vi "Dependency Change.vi"(5 "object ref in":T3, 8 "error in (no error)":errorcluster, 9 "old values":string[][](array[string]), 10 "Table Change":T2, 11 "Mapping Column in":refnum<class "Mapping Column.lvclass">) -> (0 "error out":errorcluster, 3 "Mapping Column out":refnum<class "Mapping Column.lvclass">)   [LabVIEW 2013, in "Table Manager.lvlib" / "Mapping Column.lvclass"]
uses:
  Mapping Column.lvclass
  Table Manager/object ref.ctl
  <vilib>/NI/DCAF/Tag Editor Core/Configuration Editor/Classes/Engine Parent/Engine Parent Editor Node.lvclass
  <vilib>/NI/DCAF/Tag Editor Core/Configuration Editor/Classes/Module editor node/module editor node.lvclass
  Table Manager/Cell Change.ctl
  <vilib>/NI/Tag Bus/tag/Data Type.ctl
  Mapping Column.lvclass/Mapping Column.ctl
  <vilib>/NI/Tag Bus Module Framework/module configuration/TBM module configuration.lvclass
  <vilib>/NI/Configuration Framework/serializable configuration/NISE_CEF_serializable configuration.lvclass/NISE_CEF_serializable configuration.ctl
  <vilib>/NI/Tag Bus/tag/tag descriptor.lvclass/tag descriptor.ctl
  Read Name Dependecy.vi
  Read Data Type Dependecy.vi
  Read Channel suffix.vi
  Column/Read Call Back VI.vi
  <vilib>/Utility/LVClass/Get LV Class Name.vi
  <vilib>/NI/Configuration Framework/error generator/NISE_error generator.vi
  <vilib>/NI/Module Execution Interface/Engine Configuration/engine configuration.lvclass
  <vilib>/NI/Configuration Framework/serializable configuration/NISE_CEF_serializable configuration.lvclass
  <vilib>/NI/Tag Bus/tag/tag descriptor.lvclass
  Table Manager.lvlib
  Column/Column.lvclass
  Table Manager/Table Manager.lvclass
panel:
  out "Array":string[](array[string])
  in  "data type":T1
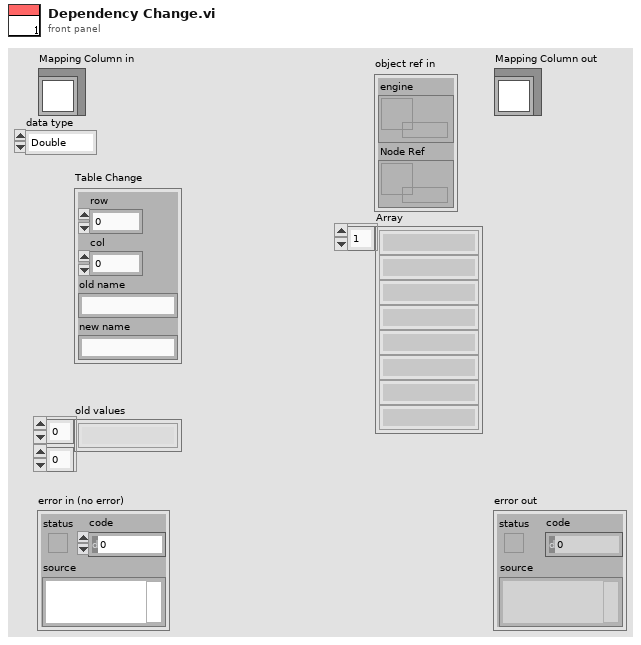
[diagram p1: front panel]
types:
  T1 = typedef "tag bus.lvlib/tag descriptor.lvclass/Data Type.ctl" = enum16{"Double", "Single", "I64", "I32", "I16", "I8", "U64", "U32", "U16", "U8", "Boolean", "String", "Array of Double", "Array of Single", "Array of I64", "Array of I32", "Array of I16", "Array of I8", "Array of U64", "Array of U32", "Array of U16", "Array of U8", "Array of Boolean", "Array of String"}
  T2 = typedef "Table Manager.lvlib/Cell Change.ctl" = cluster{"row":i32, "col":i32, "old name":string, "new name":string}
  T3 = typedef "Table Manager.lvlib/Table Manager.lvclass/object ref.ctl" = cluster{"engine":refnum<data-value>, "Node Ref":refnum<data-value>}
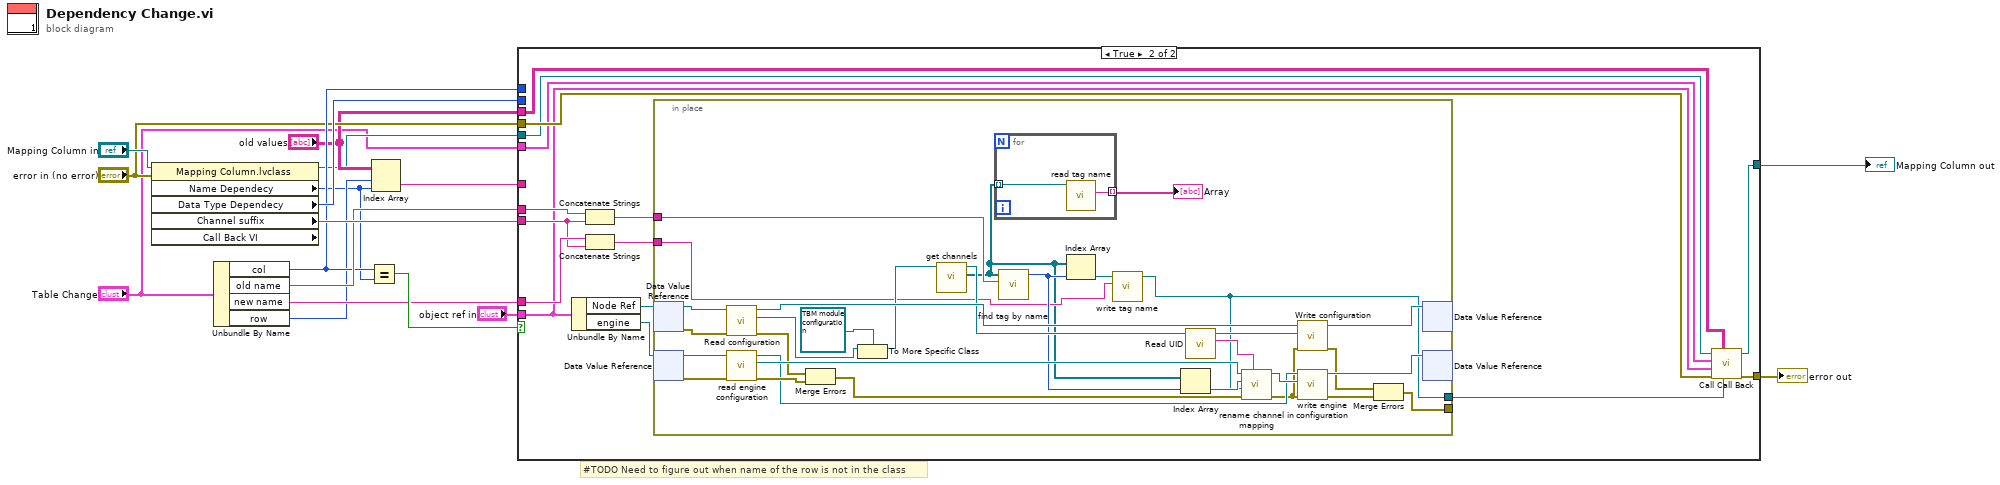
[diagram p0: block diagram]
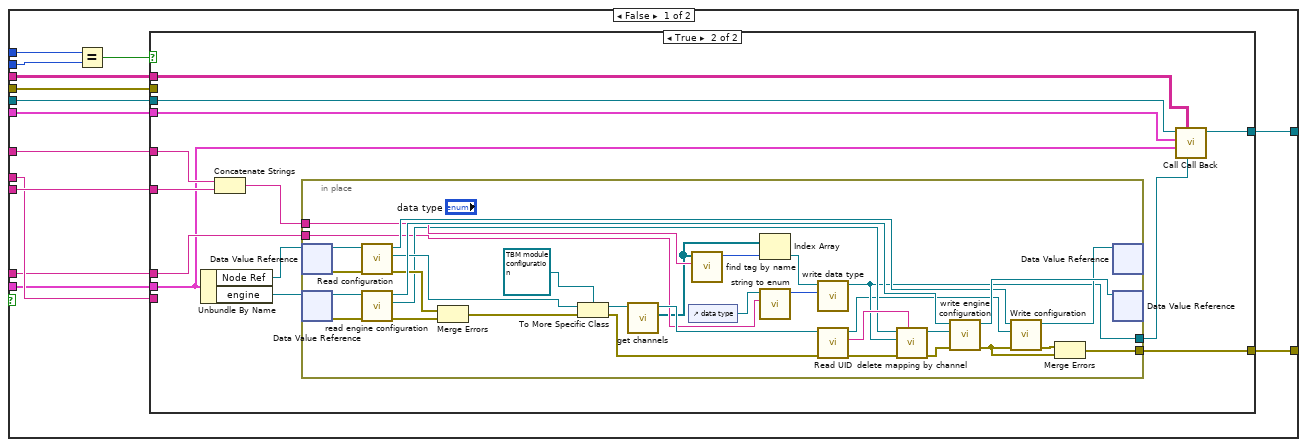
[diagram p2: hidden frame]
diagram:
  # "#TODO Need to figure out when name of the row is not in the class"
  n1 = property class="Mapping Column.lvclass" props=["Name Dependecy", "Data Type Dependecy", "Channel suffix", "Call Back VI"](reference="Mapping Column in", error in="error in (no error)") -> (reference out=w3:refnum<class "Mapping Column.lvclass">, "Name Dependecy"=w8:i32, "Data Type Dependecy"=w16:i32, "Channel suffix"=w13:string)  [unwired: 2 out]
  n2 = Unbundle By Name("Table Change") -> ("col"=w10:i32, "old name"=w12:string, "new name"=w11:string, "row"=w9:i32)
  n3 = Equal?(x=w10, y=w8) -> (x = y?=w17:bool)
  n4 = Index Array(array="old values", index (row)=w9, index (col)=w8) -> (element=w7:string)
  n5 = case shown="True" w17 {
    tunnel: w16 -> [w31 _]
    tunnel: w10 -> [w30 _]
    tunnel: "object ref in" -> [w22 w81]
    tunnel: w12 -> [w28 w91]
    tunnel: w11 -> [w27 w89]
    tunnel: w13 -> [w29 w88]
    tunnel: w7 -> [w25 _]
    tunnel: [w24 w86] -> w6
    tunnel: "error in (no error)" -> [w23 w87]
    tunnel: "old values" -> [w19 w85]
    tunnel: w3 -> [w21 w84]
    tunnel: [w20 w83] -> w2
    tunnel: "Table Change" -> [w18 w82]
    frame False {
      n6 = Equal?(x=w30, y=w31) -> (x = y?=w26:bool)
      n7 = case shown="True" w26 {
        tunnel: w22 -> [_ w34]
        tunnel: w29 -> [_ w44]
        tunnel: w28 -> [_ _]
        tunnel: w27 -> [_ w40]
        tunnel: w25 -> [_ w42]
        tunnel: [w33 w41] -> w24
        tunnel: w23 -> [w33 _]
        tunnel: w21 -> [w32 w39]
        tunnel: [w32 w38] -> w20
        tunnel: w19 -> [_ w37]
        tunnel: w18 -> [_ w36]
        frame False {
        }
        frame True {
          n8 = Unbundle By Name(w34) -> ("Node Ref"=w45:refnum<data-value>, "engine"=w46:refnum<data-value>)
          n9 = Concatenate Strings(w42, w44) -> (w43:string)
          n10 = in-place {
            in-place-border: [w72] -> w41
            in-place-border: w43 -> [w63]
            in-place-border: w40 -> [w55]
            in-place-border: [w50] -> w35
            n11 = in-place-dvr #1(w45) -> (w69:refnum<class "module editor node.lvclass">, w71:errorcluster)
            n12 = in-place-dvr #2(w46) -> (w78:refnum<class "Engine Parent Editor Node.lvclass">, w79:errorcluster)
            n13 = call-dynamic "Read configuration.vi"("error in"=w71, "NISE_CEF_serializable node in"=w69) -> ("error out"=w70:errorcluster, "configuration"=w67:refnum<class "NISE_CEF_serializable configuration.lvclass">, "NISE_CEF_serializable node out"=w68:refnum<class "module editor node.lvclass">)  [unwired: 7 in]
            n14 = call <vilib>:"read engine configuration.vi"("error in"=w79, "Engine Parent Editor Node in"=w78) -> ("error out"=w75:errorcluster, "engine configuration"=w61:refnum<class "engine configuration.lvclass">, "Engine Parent Editor Node out"=w74:refnum<class "Engine Parent Editor Node.lvclass">)  [unwired: 7 in]
            n15 = Merge Errors(w70, w75) -> (w60:errorcluster)
            n16 = To More Specific Class(target class=refnum<class "TBM module configuration.lvclass"> refnum ("module configuration"), reference=w67, error in=w60) -> (specific class reference=w65:refnum<class "TBM module configuration.lvclass">, error out=w59:errorcluster)
            n17 = call-dynamic "get channels.vi"("module configuration in"=w65) -> ("channels"=w53:refnum<class "TBM channel.lvclass">[], "module configuration out"=w64:refnum<class "TBM module configuration.lvclass">)  [unwired: 9 in]
            n18 = control-ref of="data type"() -> (w54:refnum<vi>)
            n19 = call <vilib>:"find tag by name.vi"("name"=w63, "tags in"=w53) -> ("index"=w52:i32)  [unwired: 9 in]
            n20 = Index Array(array=w53, index=w52) -> (element=w47:refnum<class "TBM channel.lvclass">)
            n21 = call "string to enum.vi"("String"=w55, "Enum"=w54) -> ("Value"=w51:i32)  [unwired: 8 in, 1 out]
            n22 = call <vilib>:"write data type.vi"("data type"=w51, "system tag in"=w47) -> ("system tag out"=w50:refnum<class "TBM channel.lvclass">)  [unwired: 8 in, 1 out]
            n23 = call <vilib>:"Read UID.vi"("error in"=w59, "configuration in"=w64) -> ("error out"=w58:errorcluster, "instance id"=w62:string, "configuration out"=w49:refnum<class "TBM module configuration.lvclass">)  [unwired: 7 in]
            n24 = call <vilib>:"delete mapping by channel.vi"("owner ID"=w62, "error in"=w58, "channel"=w50, "engine configuration in"=w61) -> ("error out"=w56:errorcluster, "engine configuration out"=w57:refnum<class "engine configuration.lvclass">)  [unwired: 6 in]
            n25 = call <vilib>:"write engine configuration.vi"("error in"=w56, "engine configuration"=w57, "Engine Parent Editor Node in"=w74) -> ("error out"=w48:errorcluster, "Engine Parent Editor Node out"=w77:refnum<class "Engine Parent Editor Node.lvclass">)  [unwired: 7 in]
            n26 = call-dynamic "Write configuration.vi"("error in"=w48, "configuration"=w49, "NISE_CEF_serializable node in"=w68) -> ("error out"=w73:errorcluster, "NISE_CEF_serializable node out"=w76:refnum<class "module editor node.lvclass">)  [unwired: 7 in]
            n27 = Merge Errors(w73, w48) -> (w72:errorcluster)
            n28 = in-place-dvr #1(w76) -> ()  [unwired: 2 out]
            n29 = in-place-dvr #2(w77) -> ()  [unwired: 2 out]
          }
          n30 = call "Call Call Back.vi"("Variant"=w35, "old values"=w37, "object ref in"=w34, "Table Change"=w36, "Column in"=w39) -> ("Column Out"=w38:refnum<class "Mapping Column.lvclass">)  [unwired: 5 in, 1 out]
        }
      }
    }
    frame True {
      n31 = Unbundle By Name(w81) -> ("Node Ref"=w93:refnum<data-value>, "engine"=w94:refnum<data-value>)
      n32 = Concatenate Strings(w91, w88) -> (w92:string)
      n33 = Concatenate Strings(w89, w88) -> (w90:string)
      n34 = in-place {
        in-place-border: [w114] -> _
        in-place-border: w92 -> [w106]
        in-place-border: w90 -> [w100]
        in-place-border: [w96] -> w80
        n35 = in-place-dvr #3(w93) -> (w111:refnum<class "module editor node.lvclass">, w113:errorcluster)
        n36 = in-place-dvr #4(w94) -> (w124:refnum<class "Engine Parent Editor Node.lvclass">, w125:errorcluster)
        n37 = call-dynamic "Read configuration.vi"("error in"=w113, "NISE_CEF_serializable node in"=w111) -> ("error out"=w112:errorcluster, "configuration"=w109:refnum<class "NISE_CEF_serializable configuration.lvclass">, "NISE_CEF_serializable node out"=w110:refnum<class "module editor node.lvclass">)  [unwired: 7 in]
        n38 = call <vilib>:"read engine configuration.vi"("error in"=w125, "Engine Parent Editor Node in"=w124) -> ("error out"=w119:errorcluster, "engine configuration"=w120:refnum<class "engine configuration.lvclass">, "Engine Parent Editor Node out"=w117:refnum<class "Engine Parent Editor Node.lvclass">)  [unwired: 7 in]
        n39 = Merge Errors(w112, w119) -> (w104:errorcluster)
        n40 = To More Specific Class(target class=refnum<class "TBM module configuration.lvclass"> refnum ("module configuration"), reference=w109) -> (specific class reference=w107:refnum<class "TBM module configuration.lvclass">)  [unwired: 1 in, 1 out]
        n41 = call-dynamic "get channels.vi"("module configuration in"=w107) -> ("channels"=w99:refnum<class "TBM channel.lvclass">[], "module configuration out"=w105:refnum<class "TBM module configuration.lvclass">)  [unwired: 9 in]
        n42 = for {
          tunnel: w99 -> [w127] mode=indexing
          tunnel: [w126] -> w98 mode=indexing
          n43 = call <vilib>:"read tag name.vi"("system tag in"=w127) -> ("name"=w126:string)  [unwired: 8 in, 2 out]
        }
        "Array" <- w98
        n44 = call <vilib>:"find tag by name.vi"("name"=w106, "tags in"=w99) -> ("index"=w102:i32)  [unwired: 9 in]
        n45 = Index Array(array=w99, index=w102) -> (element=w95:refnum<class "TBM channel.lvclass">)
        n46 = call <vilib>:"write tag name.vi"("name"=w100, "system tag in"=w95) -> ("system tag out"=w96:refnum<class "TBM channel.lvclass">)  [unwired: 8 in, 1 out]
        n47 = Index Array(array=w99, index=w102) -> (element=w101:refnum<class "TBM channel.lvclass">)
        n48 = call <vilib>:"Read UID.vi"("configuration in"=w105) -> ("instance id"=w121:string, "configuration out"=w97:refnum<class "TBM module configuration.lvclass">)  [unwired: 8 in, 1 out]
        n49 = call <vilib>:"rename channel in mapping.vi"("owner ID"=w121, "error in"=w104, "new channel"=w96, "old channel"=w101, "engine configuration in"=w120) -> ("error out"=w103:errorcluster, "engine configuration out"=w118:refnum<class "engine configuration.lvclass">)  [unwired: 5 in]
        n50 = call-dynamic "Write configuration.vi"("error in"=w103, "configuration"=w97, "NISE_CEF_serializable node in"=w110) -> ("error out"=w115:errorcluster, "NISE_CEF_serializable node out"=w122:refnum<class "module editor node.lvclass">)  [unwired: 7 in]
        n51 = call <vilib>:"write engine configuration.vi"("error in"=w103, "engine configuration"=w118, "Engine Parent Editor Node in"=w117) -> ("error out"=w116:errorcluster, "Engine Parent Editor Node out"=w123:refnum<class "Engine Parent Editor Node.lvclass">)  [unwired: 7 in]
        n52 = Merge Errors(w115, w116) -> (w114:errorcluster)
        n53 = in-place-dvr #3(w122) -> ()  [unwired: 2 out]
        n54 = in-place-dvr #4(w123) -> ()  [unwired: 2 out]
      }
      n55 = call "Call Call Back.vi"("Variant"=w80, "old values"=w85, "error in (no error)"=w87, "object ref in"=w81, "Table Change"=w82, "Column in"=w84) -> ("error out"=w86:errorcluster, "Column Out"=w83:refnum<class "Mapping Column.lvclass">)  [unwired: 4 in]
    }
  }
  "error out" <- w6
  "Mapping Column out" <- w2
